vi "CRYFind Insert Locaction in Tree Sub.vi"(7 "sAction":string, 10 "sData In":string[](array[string]), 11 "Tree In":refnum<vi>) -> (1 "ChildIndex":i32, 2 "ParentTag Out":string, 3 "Tree Out":refnum<vi>)   [LabVIEW 2013]
uses:
  CRYProject/CRYProject Editor Global.vi
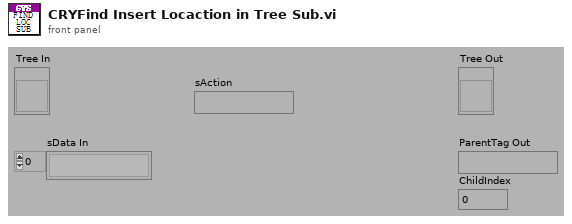
[diagram p1: front panel]
types:
  T1 = typedef "CRYStep.ctl" = cluster{"No.VI":i32, "Category":string, "StepName":string, "Seq setup flattened":string, "Comment":string, "Steps config.":bool[], "Jump config":i32[], "Start":dbl, "Increment":dbl, "Name":string, "Unit":string, "Y data":u16, "Y prefix":string, "Y dB ref":dbl, "Y unit":string, "Repeat State Array":cluster{"Start":dbl, "Increment":dbl, "Count":i32, "Num":i32}[]}
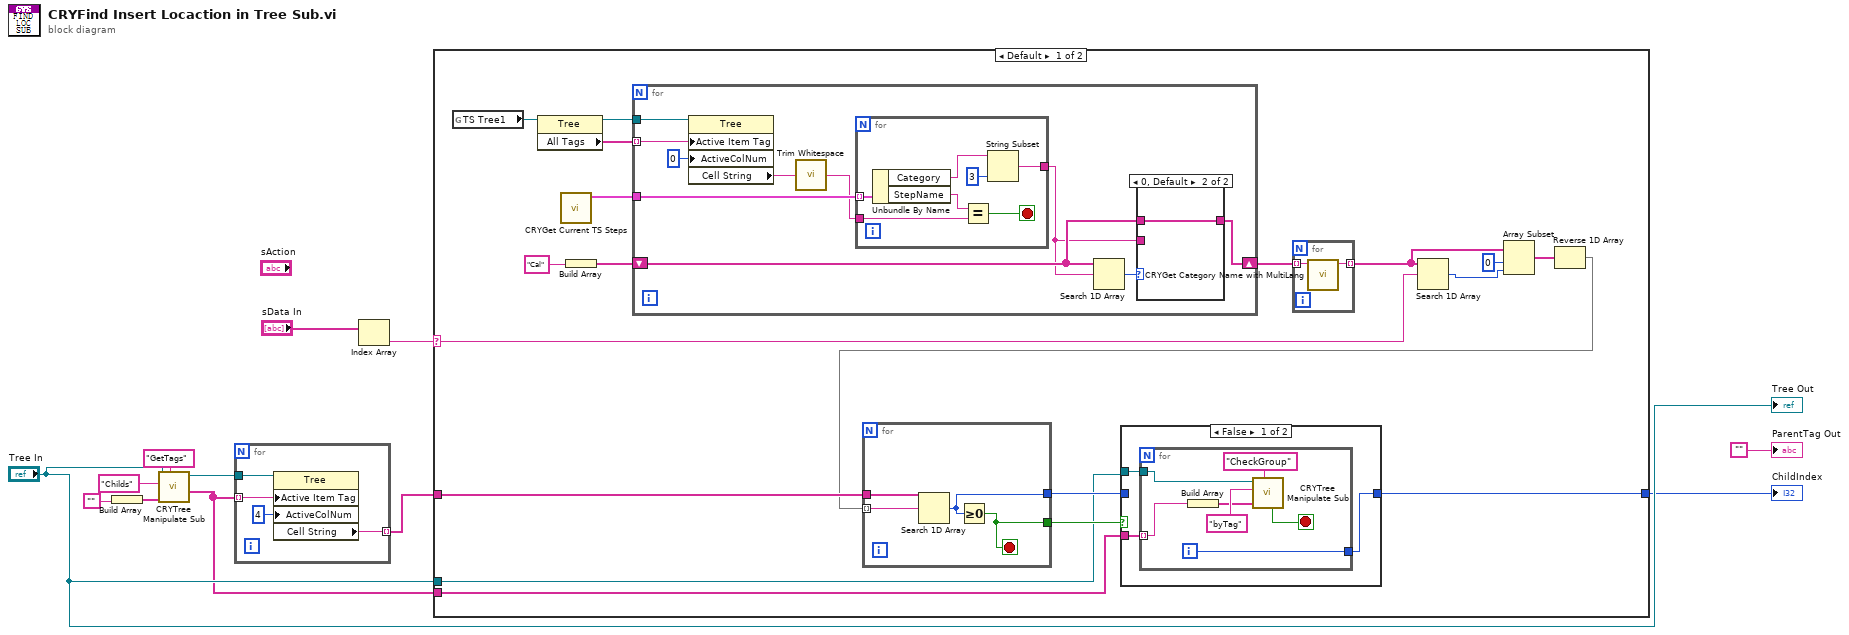
[diagram p0: block diagram]
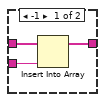
[diagram p2: hidden frame]
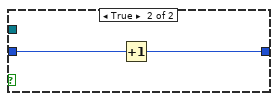
[diagram p3: hidden frame]
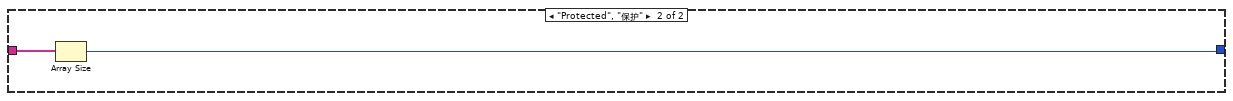
[diagram p4: hidden frame]
diagram:
  n1 = Build Array("") -> (w10:string[])
  n2 = call "CRYTree Manipulate Sub.vi"("sAction"="GetTags", "sData"=w10, "sOption"="Childs", "Tree in"="Tree In") -> ("sData Out"=w4:string[], "Tree Out"=w2:refnum<vi>)  [unwired: 3 in, 3 out]
  n3 = for {
    tunnel: w2 -> [w16]
    tunnel: w4 -> [w14] mode=indexing
    tunnel: [w13] -> w3 mode=indexing
    n4 = property class="Tree"(reference=w16, "Active Item Tag"=w14, "ActiveColNum"=4 ("Active Cell:Active Column Number")) -> ("Cell String"=w13:string)  [unwired: 1 in, 2 out]
  }
  n5 = Index Array(array="sData In") -> (element=w1:string)  [unwired: 1 in]
  n6 = case shown="Default" w1 {
    selector: w1 -> [w17 _]
    tunnel: "Tree In" -> [w33 _]
    tunnel: [w32 w75] -> w5
    tunnel: w4 -> [w31 _]
    tunnel: w3 -> [w30 w76]
    frame Default {
      n7 = global read "CRYProject Editor Global.vi" "TS Tree1"() -> (w28:refnum<vi>)
      n8 = property class="Tree"(reference=w28) -> (reference out=w27:refnum<vi>, "All Tags"=w29:string[])  [unwired: 1 in, 1 out]
      n9 = call "CRYGet Current TS Steps.vi"() -> ("Steps"=w26:T1[])  [unwired: 7 in, 4 out]
      n10 = Build Array("Cal" ("Category")) -> (w24:string[])
      n11 = for {
        tunnel: w29 -> [w48] mode=indexing
        tunnel: w27 -> [w49]
        tunnel: w26 -> [w47]
        shift-right: [w43] -> w19
        shift-left: w24 -> [w44]
        n12 = property class="Tree"(reference=w49, "Active Item Tag"=w48, "ActiveColNum"=0 ("Active Cell:Active Column Number")) -> ("Cell String"=w51:string)  [unwired: 1 in, 2 out]
        n13 = call <vilib>:"Trim Whitespace.vi"("string"=w51) -> ("trimmed string"=w46:string)  [unwired: 1 in]
        n14 = for {
          tunnel: w47 -> [w62] mode=indexing
          tunnel: w46 -> [w60]
          tunnel: [w56] -> w42
          stop <- w59 stop-if-true
          n15 = Unbundle By Name(w62) -> ("Category"=w57:string, "StepName"=w61:string)
          n16 = Equal?(x=w61, y=w60) -> (x = y?=w59:bool)
          n17 = String Subset(string=w57, length (rest)=3 ("length (rest)")) -> (substring=w56:string)  [unwired: 1 in]
        }
        n18 = Search 1D Array(1D array=w44, element=w42) -> (index of element=w45:i32)  [unwired: 1 in]
        n19 = case shown="0, Default" w45 {
          tunnel: w44 -> [w54 w55]
          tunnel: [w53 w55] -> w43
          tunnel: w42 -> [w52 _]
          frame -1 {
            n20 = Insert Into Array(array=w54, new element=w52) -> (w53:string[])  [unwired: 1 in]
          }
          frame 0, Default {
          }
        }
      }
      n21 = for {
        tunnel: w19 -> [w37] mode=indexing
        tunnel: [w36] -> w18 mode=indexing
        n22 = call "CRYGet Category Name with MultiLang.vi"("Category"=w37) -> ("Name"=w36:string)  [unwired: 10 in]
      }
      n23 = Search 1D Array(1D array=w18, element=w17) -> (index of element=w20:i32)  [unwired: 1 in]
      n24 = Array Subset(array=w18, index=0, length=w20) -> (w23:string[])
      n25 = Reverse 1D Array(array=w23) -> (reversed array=w22:string[])
      n26 = for {
        tunnel: w22 -> [w40] mode=indexing
        tunnel: w30 -> [w41]
        tunnel: [w39] -> w34
        tunnel: [w38] -> w35
        stop <- w38 stop-if-true
        n27 = Search 1D Array(1D array=w41, element=w40) -> (index of element=w39:i32)  [unwired: 1 in]
        n28 = Greater Or Equal To 0?(x=w39) -> (x >= 0?=w38:bool)
      }
      n29 = case shown="False" w35 {
        tunnel: w33 -> [w65 _]
        tunnel: w31 -> [w64 _]
        tunnel: w34 -> [_ w74]
        tunnel: [w63 w73] -> w32
        frame False {
          n30 = for {
            tunnel: [w71] -> w63
            tunnel: w65 -> [w68]
            tunnel: w64 -> [w67] mode=indexing
            i -> [w71]
            stop <- w66 stop-if-true
            n31 = Build Array(w67) -> (w69:string[])
            n32 = call "CRYTree Manipulate Sub.vi"("sAction"="CheckGroup", "sData"=w69, "sOption"="byTag", "Tree in"=w68) -> ("bCategory"=w66:bool)  [unwired: 3 in, 4 out]
          }
        }
        frame True {
          n33 = Increment(x=w74) -> (x+1=w73:i32)
        }
      }
    }
    frame "Protected", "保护" {
      n34 = Array Size(array=w76) -> (size(s)=w75:i32)
    }
  }
  "ChildIndex" <- w5
  "Tree Out" <- "Tree In"
  "ParentTag Out" <- ""
